vi "Climb_Execute.vi"() -> ()   [LabVIEW 2019]
uses:
  <vilib>/Rock Robotics/WPI/Solenoid/WPI_SolenoidValue.ctl
  Globals/Climb_Globals.vi
panel:
  out "LeadScrew_Throttle":dbl
  out "Joint_Power":dbl
  out "Pin":T1=enum."Forward"
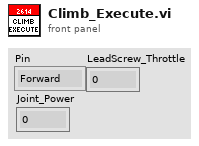
[diagram p1: front panel]
types:
  T1 = typedef "WPI_SolenoidValue.ctl" = enum16{"Off", "On", "Forward", "Reverse"}
  T2 = typedef "Climb_Cluster.ctl" = cluster{"Control_State":enum16{"No-Op", "Extending", "Clamping", "Balancing", "Manual_Control"}, "Extend_Climber?":bool, "Clamp?":bool, "Balance?":bool, "Transverse_Throttle":dbl, "Elevator_Throttle":dbl, "Control_Panel_Setpoint?":bool, "Auto-Balance":bool}
  T3 = enum16{"No-Op", "Extending", "Clamping", "Balancing", "Manual_Control"}
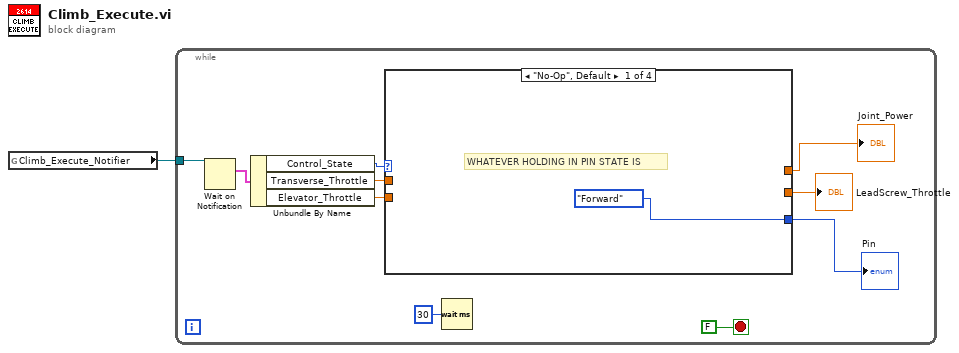
[diagram p0: block diagram]
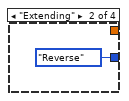
[diagram p2: hidden frame]
diagram:
  n1 = global read "Climb_Globals.vi" "Climb_Execute_Notifier"() -> (w1:refnum<notifier>)
  n2 = while {
    tunnel: w1 -> [w10]
    stop <- FALSE stop-if-true
    n3 = Wait on Notification(notifier=w10) -> (notification=w9:T2)  [unwired: 3 in, 3 out]
    n4 = Unbundle By Name(w9) -> ("Control_State"=w8:T3, "Transverse_Throttle"=w6:dbl, "Elevator_Throttle"=w4:dbl)
    n5 = case shown="\"No-Op\", Default" w8 {
      tunnel: [WPI_SolenoidValue."Forward" ("Value") WPI_SolenoidValue."Reverse" ("Value") _ _] -> w7
      tunnel: w6 -> [_ _ _ w15]
      tunnel: [_ _ _ w15] -> w5
      tunnel: w4 -> [_ _ w14 _]
      tunnel: [_ _ w14 _] -> w3
      frame "No-Op", Default {
        # "WHATEVER HOLDING IN PIN STATE IS"
      }
      frame "Extending" {
      }
      frame "Clamping" {
        # "fully manual control atm"
      }
      frame "Balancing" {
        # "all manual right now, add in auto-balance"
      }
    }
    "Pin" <- w7
    "Joint_Power" <- w5
    "LeadScrew_Throttle" <- w3
    n6 = Wait (ms)(milliseconds to wait=u32 30) -> ()  [unwired: 1 out]
  }
